vi "Test Snake Not Alive After Collission with Self.vi"(8 "error in (no error)":errorcluster, 11 "Test Case In":refnum<class "Snake Test.lvclass">) -> (0 "error out":errorcluster, 3 "Test Case Out":refnum<class "Snake Test.lvclass">)   [LabVIEW 2020, in "Snake Test.lvclass"]
uses:
  Snake Test.lvclass
  C:/Program Files (x86)/National Instruments/LabVIEW 2020/vi.lib/Astemes/LUnit/Test Case.lvclass
  source/Particle/Position.ctl
  source/Snake/Direction.ctl
  <vilib>/Astemes/LUnit/Test Case.lvclass/Test Case.ctl
  <vilib>/Astemes/LUnit/Set Assertion Type.vi
  <vilib>/Astemes/LUnit/Palette/Pass.vi
  <vilib>/Astemes/LUnit/Palette/Fail.vi
  <vilib>/Astemes/LUnit/Add test result.vi
  <vilib>/Astemes/LUnit/LUnit Record Assertion Result.vi
  <vilib>/Astemes/LUnit/LUnit Aggregate Assertion Results.vi
  <vilib>/Astemes/LUnit/Method Result/LUnit Merge Status.vi
  <vilib>/Astemes/LUnit/LUnit Concatenate result strings.vi
  source/Snake/Snake.lvclass
  source/Particle.lvclass
  <vilib>/Astemes/LUnit/Test Case.lvclass
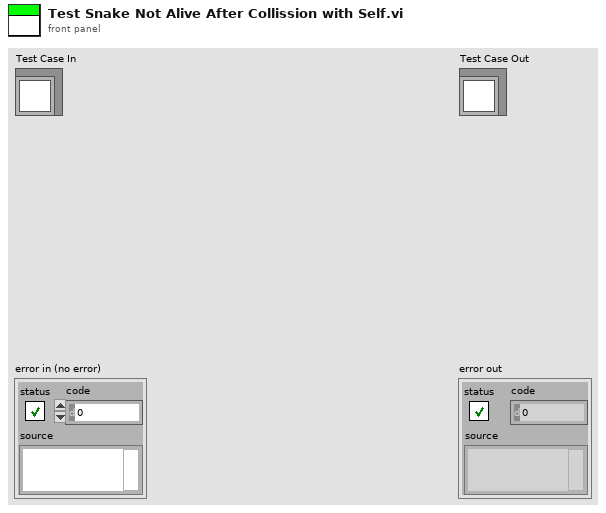
[diagram p1: front panel]
types:
  T1 = typedef "Snake.lvclass/Direction.ctl" = enum16{"X", "-X", "Y", "-Y"}
  T2 = typedef "Particle.lvclass/Position.ctl" = cluster{"X":i32, "Y":i32}
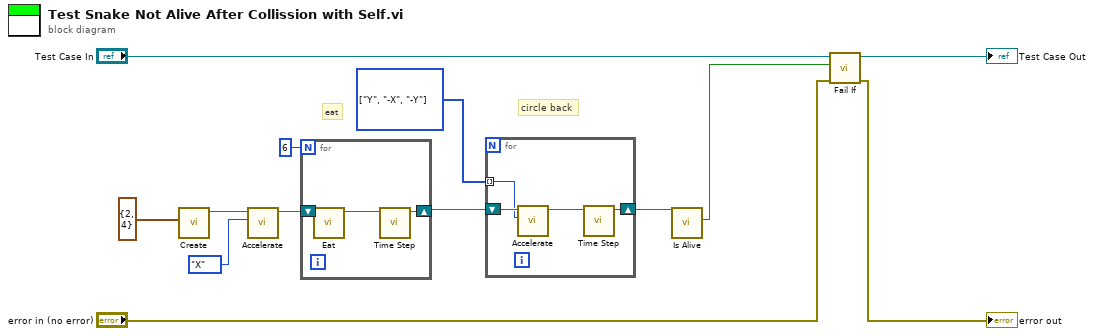
[diagram p0: block diagram]
diagram:
  w4 = T1[] [enum."Y", enum."-X", enum."-Y"] items=["X", "-X", "Y", "-Y"] ("Array")
  # "circle back"
  # "eat"
  n1 = call "Create.vi"("Position"=T2 {"X"=2, "Y"=4}) -> ("Snake out"=w9:refnum<class "Snake.lvclass">)  [unwired: 10 in]
  n2 = call "Accelerate.vi"("Direction"=enum16{"X", "-X", "Y", "-Y"}."X", "Snake in"=w9) -> ("Snake out"=w6:refnum<class "Snake.lvclass">)  [unwired: 9 in]
  n3 = for {
    N: 6 -> [_]
    shift-right: [w15] -> w3
    shift-left: w6 -> [w16]
    n4 = call "Eat.vi"("Snake in"=w16) -> ("Snake out"=w14:refnum<class "Snake.lvclass">)  [unwired: 10 in]
    n5 = call "Time Step.vi"("Snake in"=w14) -> ("Snake out"=w15:refnum<class "Snake.lvclass">)  [unwired: 10 in]
  }
  n6 = for {
    shift-right: [w19] -> w2
    shift-left: w3 -> [w20]
    tunnel: w4 -> [w17] mode=indexing
    n7 = call "Accelerate.vi"("Direction"=w17, "Snake in"=w20) -> ("Snake out"=w18:refnum<class "Snake.lvclass">)  [unwired: 9 in]
    n8 = call "Time Step.vi"("Snake in"=w18) -> ("Snake out"=w19:refnum<class "Snake.lvclass">)  [unwired: 10 in]
  }
  n9 = call "Is Alive.vi"("Snake in"=w2) -> ("Alive?"=w1:bool)  [unwired: 9 in, 1 out]
  n10 = call <vilib>:"Fail If.vi"("error in (no error)"="error in (no error)", "Fail?"=w1, "LUnit Test Case In"="Test Case In") -> ("error out"=→"error out":errorcluster, "LUnit Test Case Out"=→"Test Case Out":refnum<class "Snake Test.lvclass">)  [unwired: 7 in]
